vi "testReader.vi"() -> ()   [LabVIEW 2013]
uses:
  OCU/Location of Think.ctl
  RIO-OCU_Comm/NetworkStreams/Examples/HelperVIs/EStopAction.ctl
  RIO-OCU_Comm/NetworkStreams/Reader/NetworkStreamReader.lvclass
panel:
  out "boat speed":dbl
  out "data":i32
  in  "Loop delay (ms)":u32=10
  out "Connected?":bool
  in  "stop":bool
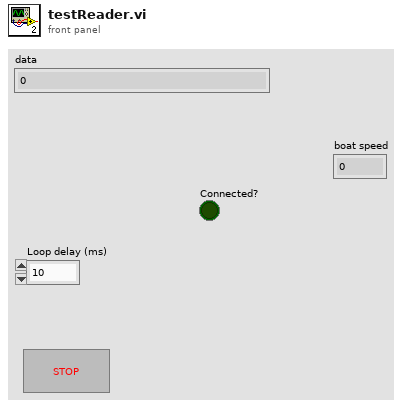
[diagram p1: front panel]
types:
  T1 = typedef "Location of Think.ctl" = string
  T2 = typedef "EStopAction.ctl" = enum16{"Get", "Set"}
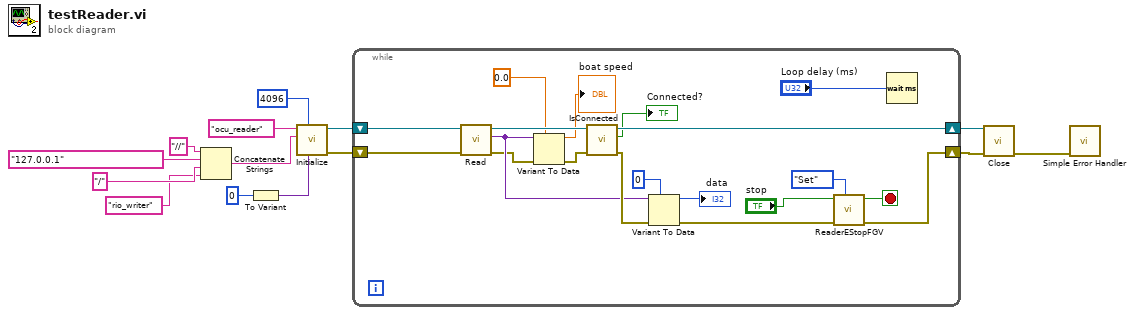
[diagram p0: block diagram]
diagram:
  n1 = Concatenate Strings("//" ("string"), T1 "127.0.0.1" ("Location of THINK"), "/", "rio_writer" ("string")) -> (w2:string)
  n2 = To Variant(anything=0) -> (Variant=w8:variant)
  n3 = call "Initialize.vi"("Default return"=w8, "reader buffer size"=4096 ("writer buffer size"), "writer url"=w2, "reader name"="ocu_reader") -> ("error out"=w14:errorcluster, "NetworkStreamReader out"=w12:refnum<class "NetworkStreamReader.lvclass">)  [unwired: 6 in]
  n4 = while {
    shift-right: [w22] -> w10
    shift-left: w12 -> [w33]
    shift-right: [w25] -> w11
    shift-left: w14 -> [w32]
    stop <- w26 stop-if-true
    n5 = call "Read.vi"("error in (no error)"=w32, "NetworkStreamReader in"=w33) -> ("error out"=w18:errorcluster, "element"=w19:variant, "NetworkStreamReader out"=w24:refnum<class "NetworkStreamReader.lvclass">)  [unwired: 5 in, 2 out]
    n6 = Variant To Data(error in=w18, type=0.0, Variant=w19) -> (data=→"boat speed":dbl, error out=w17:errorcluster)
    n7 = call "IsConnected.vi"("error in (no error)"=w17, "NetworkStreamReader in"=w24) -> ("error out"=w23:errorcluster, "Connected?"=→"Connected?":bool, "NetworkStreamReader out"=w22:refnum<class "NetworkStreamReader.lvclass">)  [unwired: 7 in]
    n8 = Variant To Data(error in=w23, type=0, Variant=w19) -> (data=→"data":i32, error out=w27:errorcluster)
    n9 = call "ReaderEStopFGV.vi"("E-Stop Action"=EStopAction."Set", "Error In"=w27, "E-Stop In"="stop") -> ("Error Out"=w25:errorcluster, "E-Stop Out"=w26:bool)  [unwired: 7 in]
    n10 = Wait (ms)(milliseconds to wait="Loop delay (ms)") -> ()  [unwired: 1 out]
  }
  n11 = call "Close.vi"("error in (no error)"=w11, "NetworkStreamReader in"=w10) -> ("error out"=w6:errorcluster)  [unwired: 9 in]
  n12 = call <vilib>:"Simple Error Handler.vi"("error in (no error)"=w6) -> ()  [unwired: 4 in, 5 out]
